vi "PythonToLabVIWImage.vi"(8 "error in (no error)":errorcluster, 10 "Python Image":u8[][][](array[numeric])) -> (0 "error out":errorcluster, 2 "LabVIEW Picture":picture)   [LabVIEW 2017, in "ImageFacialDetection.lvclass"]
doc: "converts a python 3D array image into a LabVIEW 2D picture"
uses:
  ImageFacialDetection.lvclass
  <vilib>/picture/picture.llb/imagedata.ctl
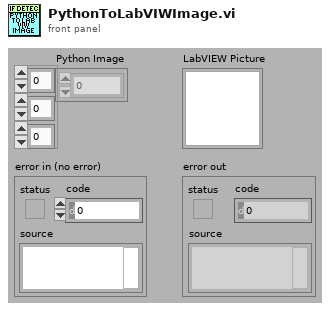
[diagram p1: front panel]
types:
  T1 = typedef "imagedata.ctl" = cluster{"image type":i32, "image depth":i32, "image":u8[], "mask":u8[], "colors":u32[], "Rectangle":cluster{"left":i16, "top":i16, "right":i16, "bottom":i16}}
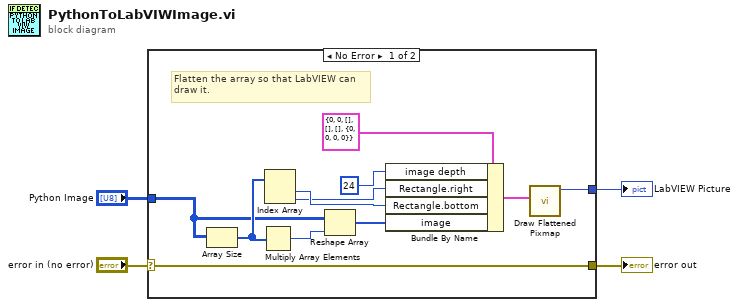
[diagram p0: block diagram]
diagram:
  n1 = case shown="No Error" "error in (no error)" {
    selector: "error in (no error)" -> [w15 w16]
    tunnel: [w15 w16] -> w3
    tunnel: "Python Image" -> [w6 _]
    tunnel: [w5 _] -> w1
    frame No Error {
      # "Flatten the array so that LabVIEW can\ndraw it."
      n2 = Array Size(array=w6) -> (size(s)=w8:i32[])
      n3 = Multiply Array Elements(1:w8) -> (0:w7:i32)
      n4 = Index Array(array=w8) -> (element #1=w11:i32, element #2=w10:i32)  [unwired: 2 in]
      n5 = Reshape Array(w6, w7) -> (w9:u8[])
      n6 = Bundle By Name(cluster=T1 {"image type"=0, "image depth"=0, "image"=[], "mask"=[], "colors"=[], "Rectangle"={"left"=0, "top"=0, "right"=0, "bottom"=0}} ("image data"), "image depth"=24, "Rectangle.right"=w10, "Rectangle.bottom"=w11, "image"=w9) -> (w12:T1)
      n7 = call <vilib>:"Draw Flattened Pixmap.vi"("image data"=w12) -> ("new picture"=w5:picture)  [unwired: 8 in]
    }
    frame Error {
    }
  }
  "error out" <- w3
  "LabVIEW Picture" <- w1
